vi "updateBathPositionsBasedOnNewStageZero_v02.vi"(8 "error in":errorcluster, 9 "preZeroStageCooridinates":i32[](array[numeric]), 11 "individual controls in":T1) -> (0 "error out":errorcluster)   [LabVIEW 2015]
uses:
  controls/memtest_def.ctl
  multipatch/controls/multipatch_individual_controls_v5.ctl
panel:
  # "Stage:"
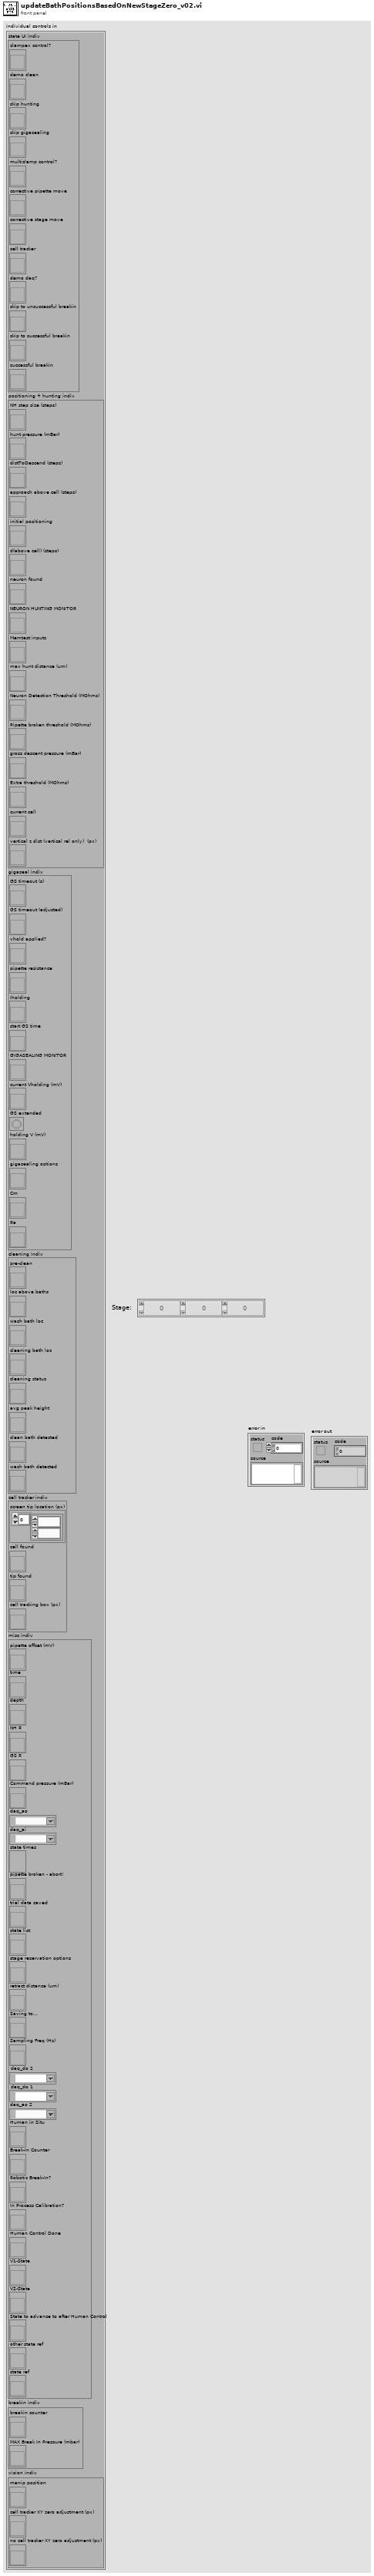
[diagram p1: front panel]
types:
  T1 = typedef "multipatch_individual_controls_v5.ctl" = cluster{"state UI indiv":cluster{"clampex control?":refnum<vi>, "demo clean":refnum<vi>, "skip hunting":refnum<vi>, "skip gigasealing":refnum<vi>, "multiclamp control?":refnum<vi>, "corrective pipette move":refnum<vi>, "corrective stage move":refnum<vi>, "cell tracker":refnum<vi>, "demo daq?":refnum<vi>, "skip to unsuccessful breakin":refnum<vi>, "skip to successful breakin":refnum<vi>, "successful breakin":refnum<vi>}, "positioning + hunting indiv":cluster{"NH step size (steps)":refnum<vi>, "hunt pressure (mBar)":refnum<vi>, "distToDescend (steps)":refnum<vi>, "approach above cell (steps)":refnum<vi>, "initial positioning":refnum<vi>, "d(above cell) (steps)":refnum<vi>, "neuron found":refnum<vi>, "NEURON HUNTING MONITOR":refnum<vi>, "Memtest inputs":refnum<vi>, "max hunt distance (um)":refnum<vi>, "Neuron Detection Threshold (MOhms)":refnum<vi>, "Pipette broken threshold (MOhms)":refnum<vi>, "gross descent pressure (mBar)":refnum<vi>, "Extra threshold (MOhms)":refnum<vi>, "current cell":refnum<vi>, "vertical z dist (vertical rel only)  (px)":refnum<vi>}, "gigaseal indiv":cluster{"GS timeout (s)":refnum<vi>, "GS timeout (adjusted)":refnum<vi>, "vhold applied?":refnum<vi>, "pipette resistance":refnum<vi>, "Iholding":refnum<vi>, "start GS time":refnum<vi>, "GIGASEALING MONITOR":refnum<vi>, "current Vholding (mV)":refnum<vi>, "GS extended":refnum<vi>, "holding V (mV)":refnum<vi>, "gigasealing options":refnum<vi>, "Cm":refnum<vi>, "Ra ":refnum<vi>}, "cleaning indiv":cluster{"pre-clean":refnum<vi>, "loc above baths":refnum<vi>, "wash bath loc":refnum<vi>, "cleaning bath loc":refnum<vi>, "cleaning status":refnum<vi>, "avg peak height":refnum<vi>, "clean bath detected":refnum<vi>, "wash bath detected":refnum<vi>}, "cell tracker indiv":cluster{"screen tip location (px)":refnum<vi>, "cell found":refnum<vi>, "tip found":refnum<vi>, "cell tracking box (px)":refnum<vi>}, "misc indiv":cluster{"pipette offset (mV)":refnum<vi>, "time":refnum<vi>, "depth":refnum<vi>, "NH R":refnum<vi>, "GS R":refnum<vi>, "Command pressure (mBar)":refnum<vi>, "daq_ao":tag, "daq_ai":tag, "state times":refnum<vi>, "pipette broken - abort!":refnum<vi>, "trial data saved":refnum<vi>, "state list":refnum<vi>, "stage reservation options":refnum<vi>, "retract distance (um)":refnum<vi>, "Saving to...":refnum<vi>, "Sampling Freq (Hz)":refnum<vi>, "daq_do 2":tag, "daq_do 1":tag, "daq_ao 2":tag, "Human in Situ":refnum<vi>, "Break-In Counter":refnum<vi>, "Robotic Break-In?":refnum<vi>, "In Process Calibration?":refnum<vi>, "Human Control Done":refnum<vi>, "V1-State":refnum<vi>, "V2-State":refnum<vi>, "State to advance to after Human Control":refnum<vi>, "other state ref":refnum<vi>, "state ref":refnum<vi>}, "breakin indiv":cluster{"breakin counter":refnum<vi>, "MAX Break In Pressure (mbar)":refnum<vi>}, "vision indiv":cluster{"manip position":refnum<vi>, "cell tracker XY zero adjustment (px)":refnum<vi>, "no cell tracker XY zero adjustment (px)":refnum<vi>}}
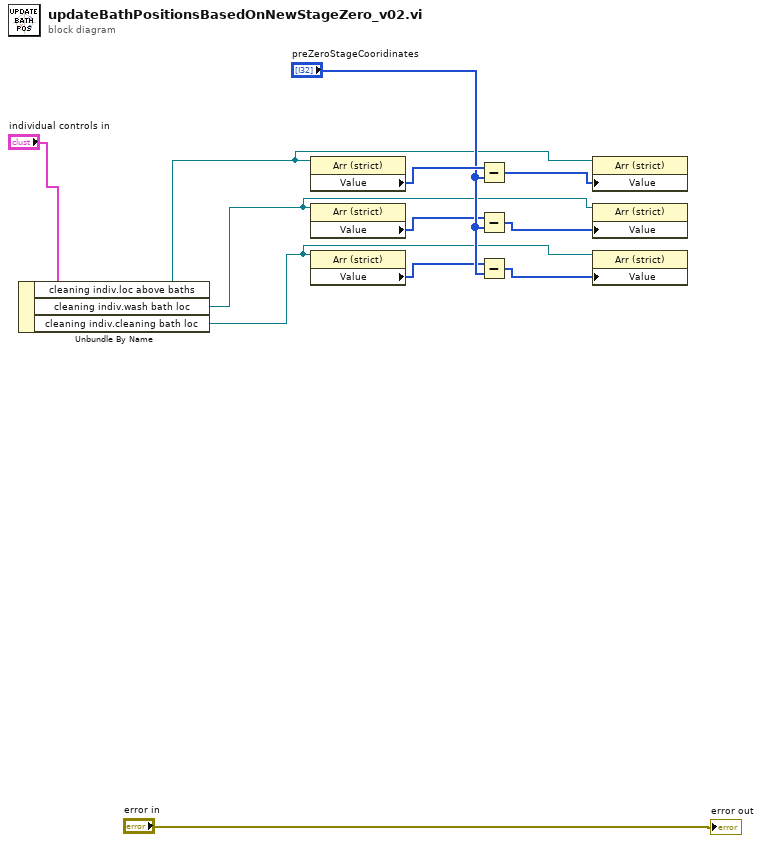
[diagram p0: block diagram]
diagram:
  n1 = Unbundle By Name("individual controls in") -> ("cleaning indiv.loc above baths"=w7:refnum<vi>, "cleaning indiv.wash bath loc"=w6:refnum<vi>, "cleaning indiv.cleaning bath loc"=w5:refnum<vi>)
  n2 = property class="Arr (strict)"(reference=w7) -> ("Value"=w12:i32[])  [unwired: 1 in, 2 out]
  n3 = property class="Arr (strict)"(reference=w6) -> ("Value"=w9:i32[])  [unwired: 1 in, 2 out]
  n4 = property class="Arr (strict)"(reference=w5) -> ("Value"=w4:i32[])  [unwired: 1 in, 2 out]
  n5 = Subtract(x=w12, y="preZeroStageCooridinates") -> (x-y=w11:i32[])
  n6 = Subtract(x=w9, y="preZeroStageCooridinates") -> (x-y=w8:i32[])
  n7 = Subtract(x=w4, y="preZeroStageCooridinates") -> (x-y=w3:i32[])
  n8 = property class="Arr (strict)"(reference=w7, "Value"=w11) -> ()  [unwired: 1 in, 2 out]
  n9 = property class="Arr (strict)"(reference=w6, "Value"=w8) -> ()  [unwired: 1 in, 2 out]
  n10 = property class="Arr (strict)"(reference=w5, "Value"=w3) -> ()  [unwired: 1 in, 2 out]
  "error out" <- "error in"
